vi "Sequencer test.vi"() -> ()   [LabVIEW 2020]
uses:
  PPL/HDH.Actor Framework.Core.Publisher.lvlibp/Publisher/Publisher.lvclass
  C:/Current projects/WS/PPL/HDH.Actor Framework.Core.Actor.lvlibp/1abvi3w/vi.lib/ActorFramework/Actor/Actor.lvclass
  Actor/Dummy Actor/Dummy Actor.lvclass
  PPL/HDH.Actor Framework.Core.Sequencer.lvlibp/Sequencer/Sequencer.lvclass
  PPL/HDH.Actor Framework.Core.Sequencer.lvlibp/Sequencer Messages/Cycle Msg/Cycle Msg.lvclass
  C:/Current projects/WS/PPL/HDH.Actor Framework.Core.Sequencer.lvlibp/Sequencer Messages/Sequencer Msg/Sequencer Msg.lvclass
  PPL/HDH.Actor Framework.Core.Sequencer.lvlibp/Sequencer Messages/Interrupt Sequncer Msg/Interrupt Sequncer Msg.lvclass
  PPL/HDH.Actor Framework.Core.Sequencer.lvlibp/Sequencer Messages/Flush Sequncer Msg/Flush Sequncer Msg.lvclass
  C:/Current projects/WS/PPL/HDH.Actor Framework.Core.Actor.lvlibp/1abvi3w/vi.lib/ActorFramework/Message/Message.lvclass
  PPL/HDH.Actor Framework.Core.Sequencer.lvlibp/Sequencer Messages/Wait Msg/Wait Msg.lvclass
  PPL/HDH.Actor Framework.Core.Sequencer.lvlibp/Sequencer Messages/Sequencer Msg/Sequencer Msg.lvclass
  PPL/HDH.Actor Framework.Core.Publisher.lvlibp/Publisher Messages/Targetted Msg/Targetted Msg.lvclass
  PPL/HDH.Actor Framework.Core.Actor.lvlibp/1abvi3w/vi.lib/ActorFramework/Actor/Actor.lvclass
  PPL/HDH.Actor Framework.Core.Publisher.lvlibp/Publisher Messages/Launch Subscriber Msg/Launch Subscriber Msg.lvclass
  PPL/HDH.Actor Framework.Core.Actor.lvlibp
  PPL/HDH.Actor Framework.Core.Actor.lvlibp/1abvi3w/vi.lib/ActorFramework/Stop Msg/Stop Msg.lvclass
  PPL/HDH.Actor Framework.Core.Sequencer.lvlibp/Sequencer Messages/Batch Msg/Batch Msg.lvclass
  C:/Current projects/WS/PPL/HDH.Actor Framework.Core.Sequencer.lvlibp/Sequencer Messages/Batch Msg/Batch Msg.lvclass
panel:
  in  "Flush":bool
  in  "stop":bool
  out "error out":errorcluster
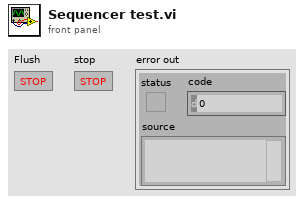
[diagram p1: front panel]
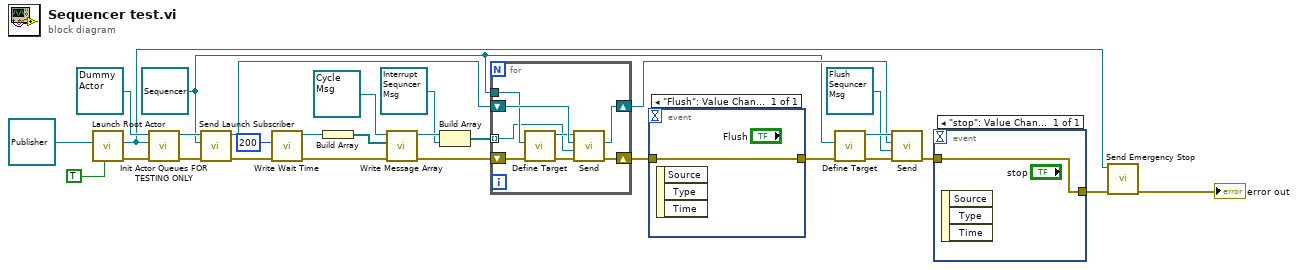
[diagram p0: block diagram]
diagram:
  w4 = refnum<class "Sequencer.lvclass"> refnum ("HDH.Actor Framework.Core.Sequencer.lvlibp:Sequencer.lvclass")
  n1 = call "Launch Root Actor.vi"("Open Actor Core front panel? (F)"=TRUE, "Actor"=refnum<class "Publisher.lvclass"> refnum ("HDH.Actor Framework.Core.Publisher.lvlibp:Publisher.lvclass")) -> ("error out"=w24:errorcluster, "Actor's Enqueuer"=w9:refnum<class "Message Enqueuer.lvclass">)  [unwired: 8 in]
  n2 = call "Init Actor Queues FOR TESTING ONLY.vi"("error in (no error)"=w24, "Actor-To-Caller Enqueuer"=w9, "Actor in"=refnum<class "Dummy Actor.lvclass"> refnum ("Test Actor.lvlib:Test Actor.lvclass")) -> ("error out"=w23:errorcluster, "Actor out"=w26:refnum<class "Dummy Actor.lvclass">)  [unwired: 5 in, 2 out]
  n3 = call "Send Launch Subscriber.vi"("error in (no error)"=w23, "Actor to Launch"=w4, "Actor in"=w26) -> ("error out"=w16:errorcluster, "Actor out"=w8:refnum<class "Dummy Actor.lvclass">)  [unwired: 6 in, 1 out]
  n4 = call "Write Wait Time.vi"("error in (no error)"=w16, "Wait Time in ms (0)"=200) -> ("error out"=w19:errorcluster, "Wait Msg out"=w21:refnum<class "Wait Msg.lvclass">)  [unwired: 8 in]
  n5 = Build Array(w21) -> (w20:refnum<class "Wait Msg.lvclass">[])
  n6 = call "Write Message Array.vi"("error in (no error)"=w19, "Message Array"=w20, "Batch Msg in"=refnum<class "Cycle Msg.lvclass"> refnum ("HDH.Actor Framework.Core.Sequencer.lvlibp:Cycle Msg.lvclass")) -> ("error out"=w15:errorcluster, "Batch Msg out"=w17:refnum<class "Cycle Msg.lvclass">)  [unwired: 7 in]
  n7 = Build Array(w17, refnum<class "Interrupt Sequncer Msg.lvclass"> refnum ("HDH.Actor Framework.Core.Sequencer.lvlibp:Interrupt Sequncer Msg.lvclass")) -> (w12:refnum<class "Sequencer Msg.lvclass">[])
  n8 = for {
    tunnel: w4 -> [w34]
    tunnel: w12 -> [w30] mode=indexing
    shift-right: [w35] -> w10
    shift-left: w15 -> [w32]
    shift-right: [w29] -> w6
    shift-left: w8 -> [w36]
    n9 = call "Define Target.vi"("error in (no error)"=w32, "Target Actor"=w34) -> ("error out"=w31:errorcluster, "Targetted Msg out"=w33:refnum<class "Targetted Msg.lvclass">)  [unwired: 8 in]
    n10 = call-dynamic "Send.vi"("error in (no error)"=w31, "Message"=w30, "Actor in"=w36, "Targetted Msg in"=w33) -> ("error out"=w35:errorcluster, "Actor out"=w29:refnum<class "Actor.lvclass">)  [unwired: 5 in, 1 out]
  }
  n11 = event shown="[0] \"Flush\": Value Change" {
    selector: _ -> [_]
    dyn-events: _ -> [_]
    timeout: _ -> [_]
    tunnel: [w37] -> w3
    tunnel: w10 -> [w37]
    event "Flush": Value Change {
      n12 = event-data() -> ()  [unwired: 1 in, 3 out]
    }
  }
  n13 = call "Define Target.vi"("error in (no error)"=w3, "Target Actor"=w4) -> ("error out"=w2:errorcluster, "Targetted Msg out"=w7:refnum<class "Targetted Msg.lvclass">)  [unwired: 8 in]
  n14 = call-dynamic "Send.vi"("error in (no error)"=w2, "Message"=refnum<class "Flush Sequncer Msg.lvclass"> refnum ("HDH.Actor Framework.Core.Sequencer.lvlibp:Flush Sequncer Msg.lvclass"), "Actor in"=w6, "Targetted Msg in"=w7) -> ("error out"=w1:errorcluster)  [unwired: 5 in, 2 out]
  n15 = event shown="[0] \"stop\": Value Change" {
    selector: _ -> [_]
    dyn-events: _ -> [_]
    timeout: _ -> [_]
    tunnel: [w38] -> w14
    tunnel: w1 -> [w38]
    event "stop": Value Change {
      n16 = event-data() -> ()  [unwired: 1 in, 3 out]
    }
  }
  n17 = call "Send Emergency Stop.vi"("error in (no error)"=w14, "Message Enqueuer"=w9) -> ("error out"=→"error out":errorcluster)  [unwired: 9 in]
